vi "glueing_recovery.vi"() -> ()   [LabVIEW 2011]
panel:
  in  "OK Button 2":bool
  in  "Y to be glued (mm)":dbl
  in  "X to be glued (mm)":dbl
  in  "OK Button":bool
  in  "Motor":u16(ring) items=["X", "Y", "Z", "Gluer", "Spint"]
  in  "mm":dbl
  in  "KILL":bool
  in  "PAUSE":bool
  in  "RESUME":bool
  in  "QUIT":bool
  in  "zero Spint":bool
  out "output":string
  out "command":string
  in  "zero Gluer":bool
  in  "zero x":bool
  in  "zero y":bool
  # "Posiziono in zero"
  # "Movimentazione Motori"
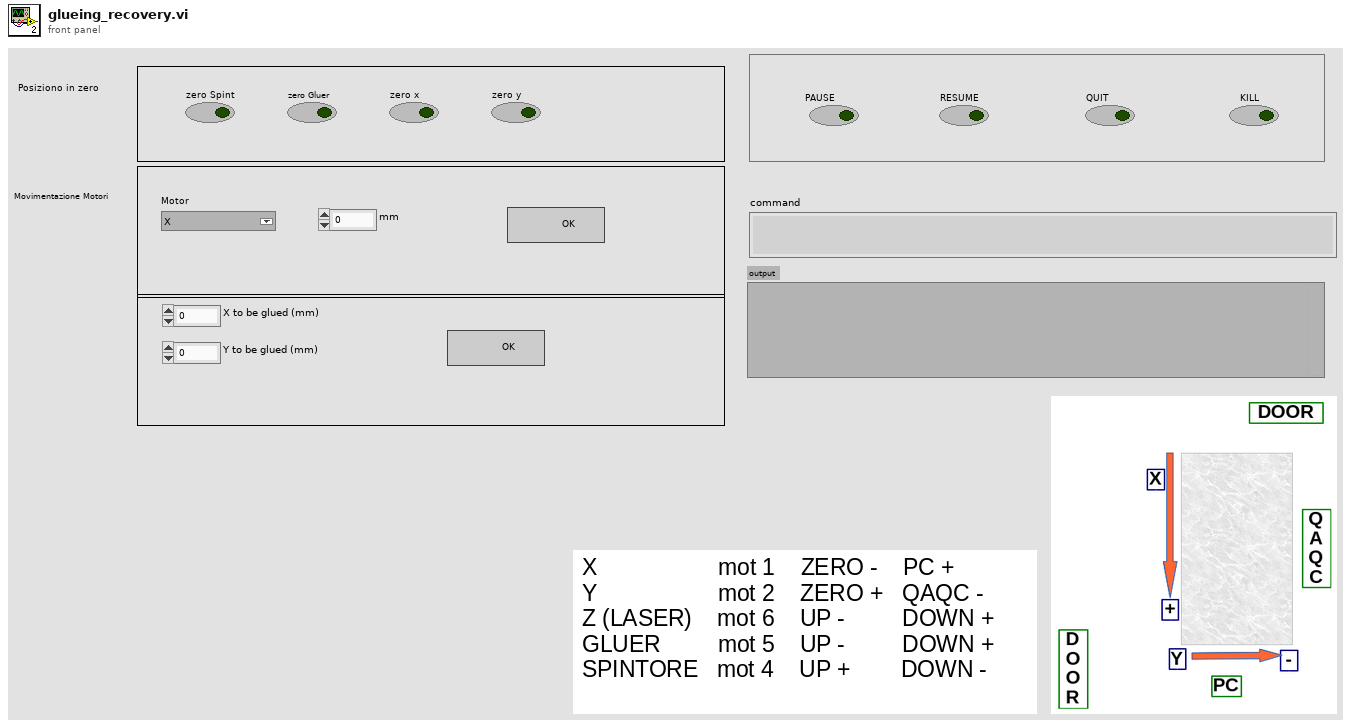
[diagram p1: front panel]
types:
  T1 = enum16{"open", "replace", "create", "open or create", "replace or create", "replace or create with confirmation"}
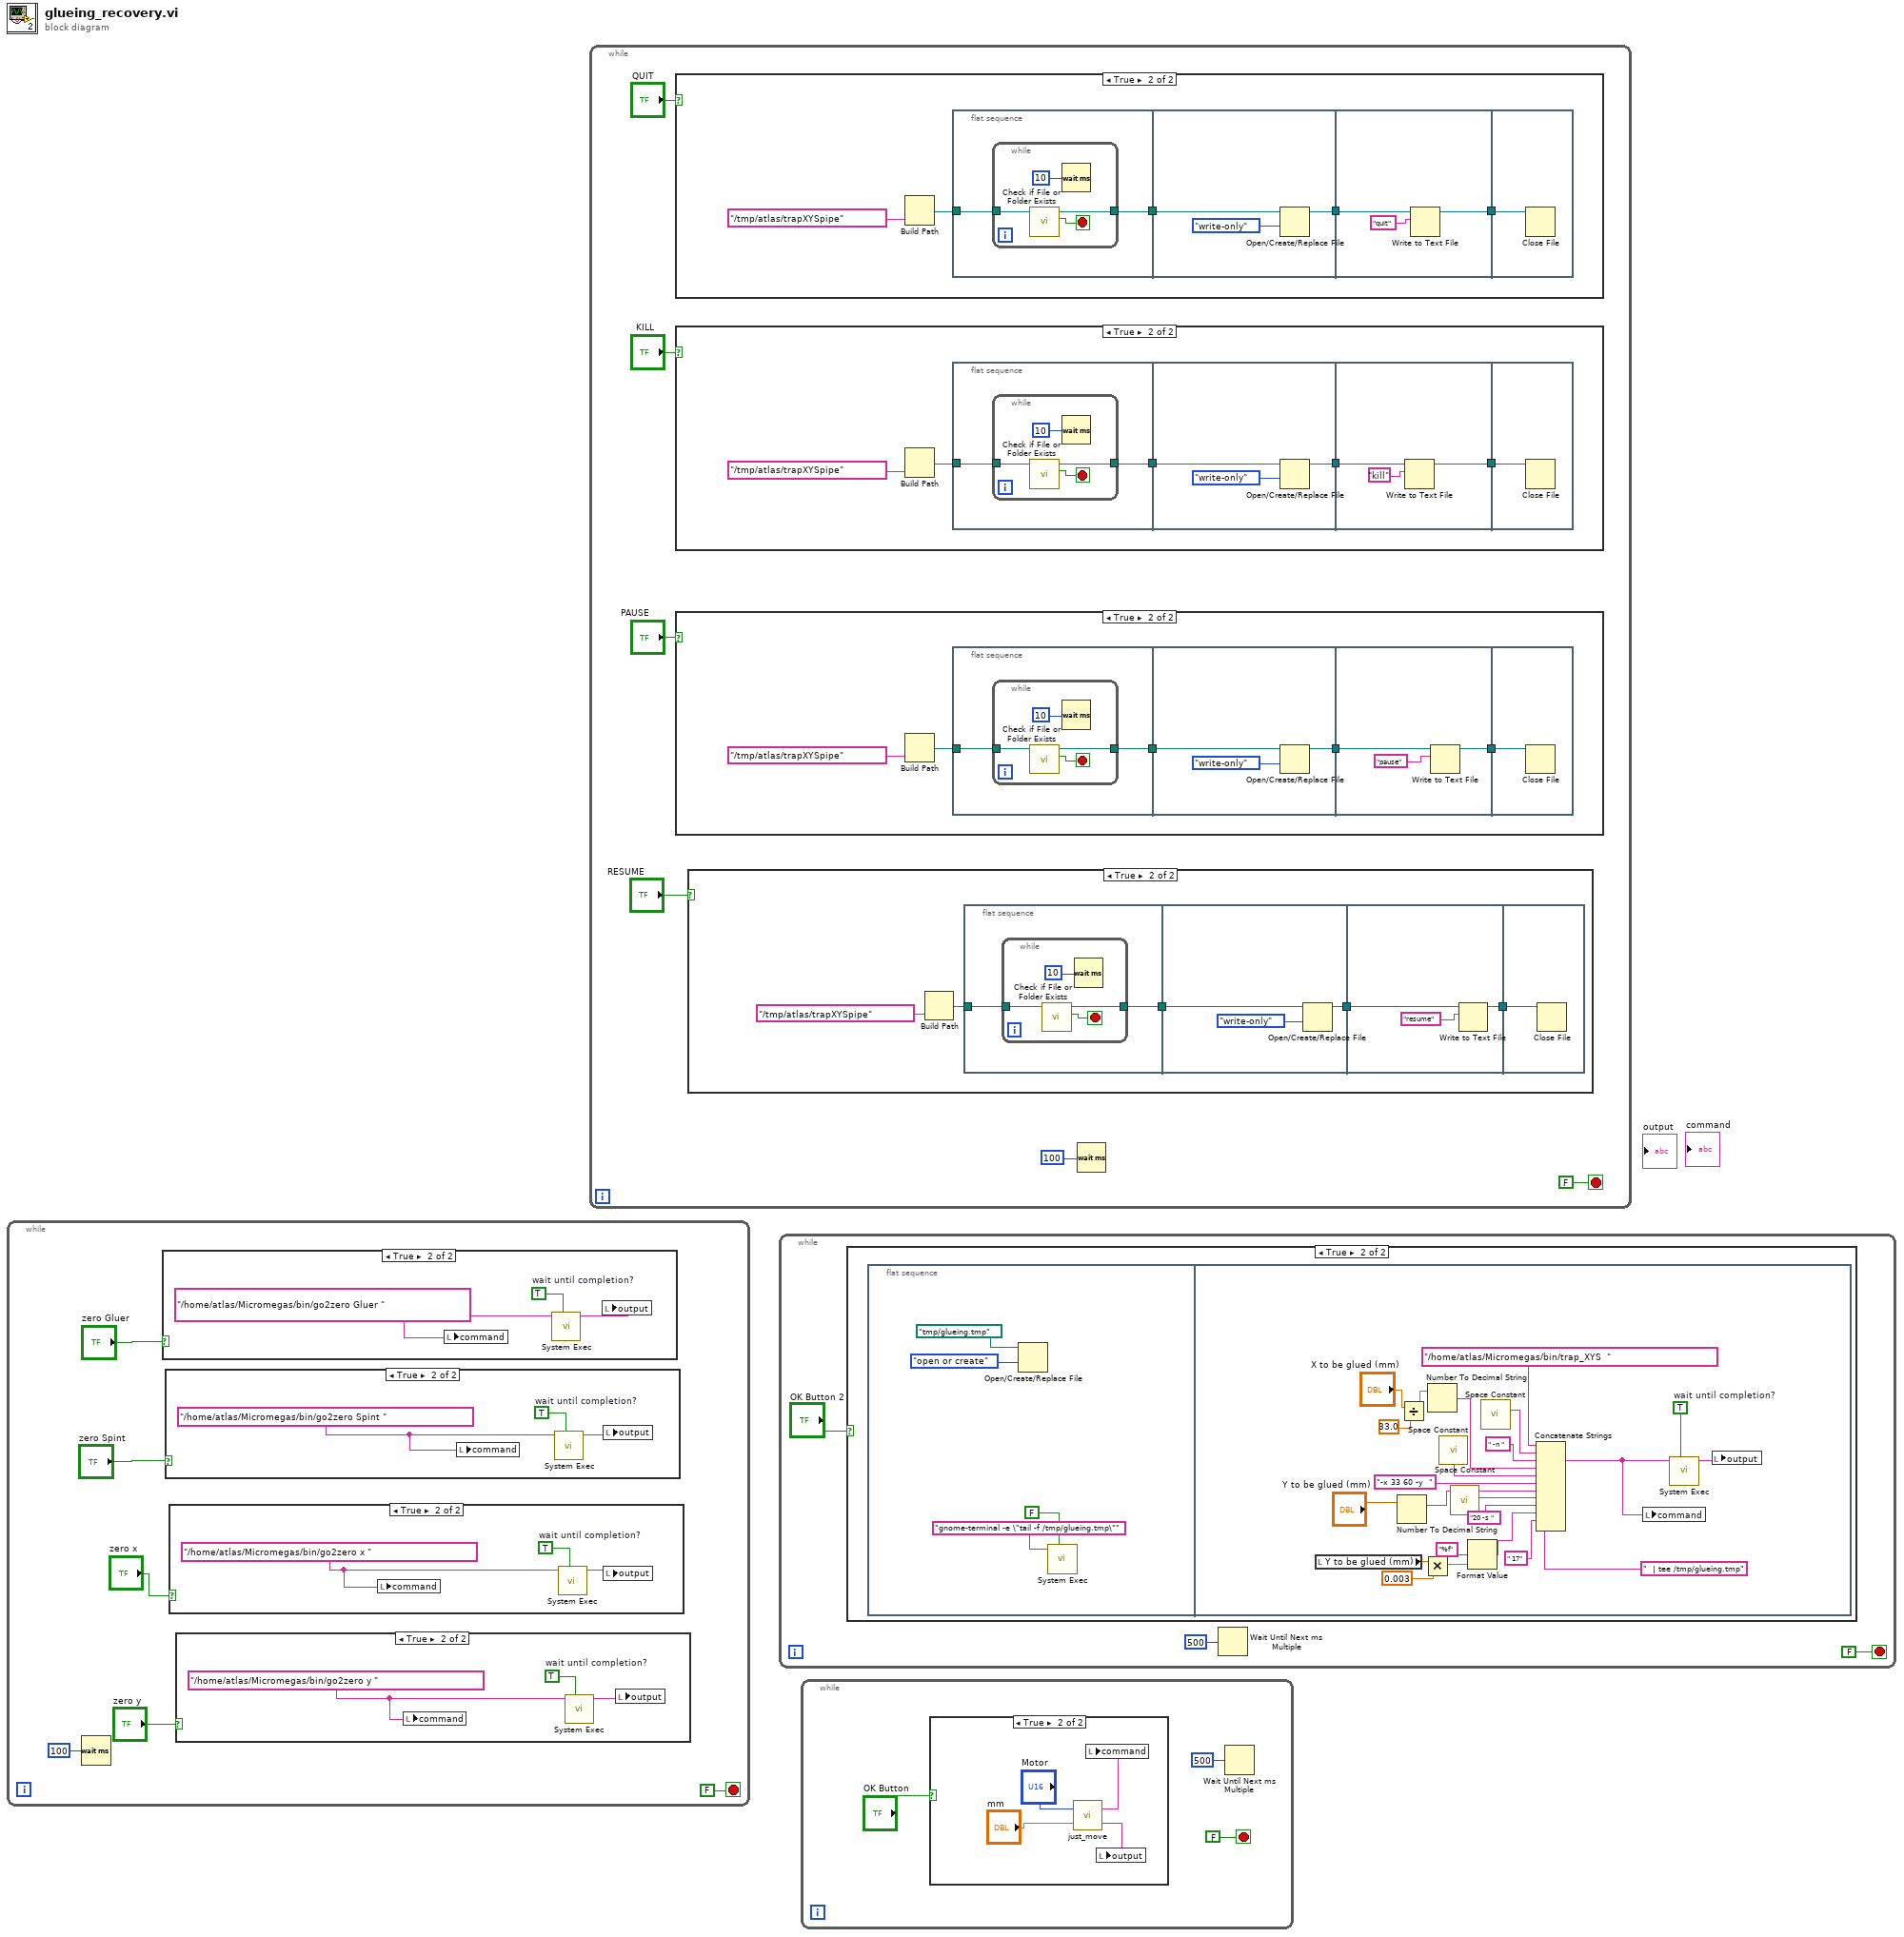
[diagram p0: block diagram]
diagram:
  n1 = while {
    stop <- FALSE stop-if-true
    n2 = Wait (ms)(milliseconds to wait=u32 100) -> ()  [unwired: 1 out]
    n3 = case shown="True" "zero Gluer" {
      frame False {
      }
      frame True {
        w17 = "/home/atlas/Micromegas/bin/go2zero Gluer " ("string")
        w18 = TRUE  # wait until completion?
        n4 = local write "command"(w17) -> ()
        n5 = call <vilib>:"System Exec.vi"("wait until completion? (T)"=w18, "command line"=w17) -> ("standard output"=w16:string)  [unwired: 6 in, 3 out]
        n6 = local write "output"(w16) -> ()
      }
    }
    n7 = case shown="True" "zero Spint" {
      frame False {
      }
      frame True {
        w7 = "/home/atlas/Micromegas/bin/go2zero Spint " ("string")
        w9 = TRUE  # wait until completion?
        n8 = local write "command"(w7) -> ()
        n9 = call <vilib>:"System Exec.vi"("wait until completion? (T)"=w9, "command line"=w7) -> ("standard output"=w8:string)  [unwired: 6 in, 3 out]
        n10 = local write "output"(w8) -> ()
      }
    }
    n11 = case shown="True" "zero x" {
      frame False {
      }
      frame True {
        w14 = "/home/atlas/Micromegas/bin/go2zero x " ("string")
        w15 = TRUE  # wait until completion?
        n12 = local write "command"(w14) -> ()
        n13 = call <vilib>:"System Exec.vi"("wait until completion? (T)"=w15, "command line"=w14) -> ("standard output"=w13:string)  [unwired: 6 in, 3 out]
        n14 = local write "output"(w13) -> ()
      }
    }
    n15 = case shown="True" "zero y" {
      frame False {
      }
      frame True {
        w11 = "/home/atlas/Micromegas/bin/go2zero y " ("string")
        w12 = TRUE  # wait until completion?
        n16 = local write "command"(w11) -> ()
        n17 = call <vilib>:"System Exec.vi"("wait until completion? (T)"=w12, "command line"=w11) -> ("standard output"=w10:string)  [unwired: 6 in, 3 out]
        n18 = local write "output"(w10) -> ()
      }
    }
  }
  n19 = while {
    stop <- FALSE stop-if-true
    n20 = case shown="True" "QUIT" {
      frame False {
      }
      frame True {
        n21 = Build Path(name or relative path="/tmp/atlas/trapXYSpipe" ("string")) -> (appended path=w79:path)  [unwired: 1 in]
        n22 = flat-sequence {
          tunnel: [w85] -> w83
          tunnel: w79 -> [w84]
          tunnel: w83 -> [w92]
          tunnel: [w90] -> w82
          tunnel: w82 -> [w95]
          tunnel: [w94] -> w81
          tunnel: w81 -> [w96]
          frame #0 {
            n23 = while {
              tunnel: [w87] -> w85
              tunnel: w84 -> [w86]
              stop <- w88 stop-if-true
              n24 = call <vilib>:"Check if File or Folder Exists.vi"("path"=w86) -> ("file or folder exists?"=w88:bool, "dup path"=w87:path)  [unwired: 8 in, 1 out]
              n25 = Wait (ms)(milliseconds to wait=u32 10) -> ()  [unwired: 1 out]
            }
          }
          frame #1 {
            n26 = Open/Create/Replace File(file path (use dialog)=w92, access (0:read/write)=enum16{"read/write", "read-only", "write-only"}."write-only") -> (refnum out=w90:refnum<file>)  [unwired: 4 in, 2 out]
          }
          frame #2 {
            n27 = Write to Text File(file (use dialog)=w95, text="quit") -> (refnum out=w94:refnum<file>)  [unwired: 2 in, 2 out]
          }
          frame #3 {
            n28 = Close File(refnum=w96) -> ()  [unwired: 1 in, 2 out]
          }
        }
      }
    }
    n29 = case shown="True" "KILL" {
      frame False {
      }
      frame True {
        n30 = Build Path(name or relative path="/tmp/atlas/trapXYSpipe" ("string")) -> (appended path=w43:path)  [unwired: 1 in]
        n31 = flat-sequence {
          tunnel: [w49] -> w47
          tunnel: w43 -> [w48]
          tunnel: w47 -> [w56]
          tunnel: [w54] -> w46
          tunnel: w46 -> [w59]
          tunnel: [w58] -> w45
          tunnel: w45 -> [w60]
          frame #0 {
            n32 = while {
              tunnel: [w51] -> w49
              tunnel: w48 -> [w50]
              stop <- w52 stop-if-true
              n33 = call <vilib>:"Check if File or Folder Exists.vi"("path"=w50) -> ("file or folder exists?"=w52:bool, "dup path"=w51:path)  [unwired: 8 in, 1 out]
              n34 = Wait (ms)(milliseconds to wait=u32 10) -> ()  [unwired: 1 out]
            }
          }
          frame #1 {
            n35 = Open/Create/Replace File(file path (use dialog)=w56, access (0:read/write)=enum16{"read/write", "read-only", "write-only"}."write-only") -> (refnum out=w54:refnum<file>)  [unwired: 4 in, 2 out]
          }
          frame #2 {
            n36 = Write to Text File(file (use dialog)=w59, text="kill") -> (refnum out=w58:refnum<file>)  [unwired: 2 in, 2 out]
          }
          frame #3 {
            n37 = Close File(refnum=w60) -> ()  [unwired: 1 in, 2 out]
          }
        }
      }
    }
    n38 = case shown="True" "PAUSE" {
      frame False {
      }
      frame True {
        n39 = Build Path(name or relative path="/tmp/atlas/trapXYSpipe" ("string")) -> (appended path=w25:path)  [unwired: 1 in]
        n40 = flat-sequence {
          tunnel: [w31] -> w29
          tunnel: w25 -> [w30]
          tunnel: w29 -> [w38]
          tunnel: [w36] -> w28
          tunnel: w28 -> [w41]
          tunnel: [w40] -> w27
          tunnel: w27 -> [w42]
          frame #0 {
            n41 = while {
              tunnel: [w33] -> w31
              tunnel: w30 -> [w32]
              stop <- w34 stop-if-true
              n42 = call <vilib>:"Check if File or Folder Exists.vi"("path"=w32) -> ("file or folder exists?"=w34:bool, "dup path"=w33:path)  [unwired: 8 in, 1 out]
              n43 = Wait (ms)(milliseconds to wait=u32 10) -> ()  [unwired: 1 out]
            }
          }
          frame #1 {
            n44 = Open/Create/Replace File(file path (use dialog)=w38, access (0:read/write)=enum16{"read/write", "read-only", "write-only"}."write-only") -> (refnum out=w36:refnum<file>)  [unwired: 4 in, 2 out]
          }
          frame #2 {
            n45 = Write to Text File(file (use dialog)=w41, text="pause") -> (refnum out=w40:refnum<file>)  [unwired: 2 in, 2 out]
          }
          frame #3 {
            n46 = Close File(refnum=w42) -> ()  [unwired: 1 in, 2 out]
          }
        }
      }
    }
    n47 = case shown="True" "RESUME" {
      frame False {
      }
      frame True {
        n48 = Build Path(name or relative path="/tmp/atlas/trapXYSpipe" ("string")) -> (appended path=w61:path)  [unwired: 1 in]
        n49 = flat-sequence {
          tunnel: [w67] -> w65
          tunnel: w61 -> [w66]
          tunnel: w65 -> [w74]
          tunnel: [w72] -> w64
          tunnel: w64 -> [w77]
          tunnel: [w76] -> w63
          tunnel: w63 -> [w78]
          frame #0 {
            n50 = while {
              tunnel: [w69] -> w67
              tunnel: w66 -> [w68]
              stop <- w70 stop-if-true
              n51 = call <vilib>:"Check if File or Folder Exists.vi"("path"=w68) -> ("file or folder exists?"=w70:bool, "dup path"=w69:path)  [unwired: 8 in, 1 out]
              n52 = Wait (ms)(milliseconds to wait=u32 10) -> ()  [unwired: 1 out]
            }
          }
          frame #1 {
            n53 = Open/Create/Replace File(file path (use dialog)=w74, access (0:read/write)=enum16{"read/write", "read-only", "write-only"}."write-only") -> (refnum out=w72:refnum<file>)  [unwired: 4 in, 2 out]
          }
          frame #2 {
            n54 = Write to Text File(file (use dialog)=w77, text="resume") -> (refnum out=w76:refnum<file>)  [unwired: 2 in, 2 out]
          }
          frame #3 {
            n55 = Close File(refnum=w78) -> ()  [unwired: 1 in, 2 out]
          }
        }
      }
    }
    n56 = Wait (ms)(milliseconds to wait=100) -> ()  [unwired: 1 out]
  }
  n57 = while {
    stop <- FALSE stop-if-true
    n58 = case shown="True" "OK Button 2" {
      frame False {
      }
      frame True {
        n59 = flat-sequence {
          frame #0 {
            n60 = Open/Create/Replace File(file path (use dialog)=path "/tmp/glueing.tmp", operation (0:open)=T1."open or create") -> ()  [unwired: 4 in, 3 out]
            n61 = call <vilib>:"System Exec.vi"("wait until completion? (T)"=FALSE, "command line"="gnome-terminal -e \"tail -f /tmp/glueing.tmp\"" ("logwindow")) -> ()  [unwired: 6 in, 4 out]
          }
          frame #1 {
            w126 = TRUE  # wait until completion?
            n62 = local read "Y to be glued (mm)"() -> (w112:dbl)
            n63 = Number To Decimal String(number="Y to be glued (mm)") -> (decimal integer string=w108:string)  [unwired: 1 in]
            n64 = Divide(x="X to be glued (mm)", y=33.0) -> (x/y=w106:dbl)
            n65 = Multiply(x=w112, y=0.003) -> (x*y=w109:dbl)
            n66 = Number To Decimal String(number=w106) -> (decimal integer string=w105:string)  [unwired: 1 in]
            n67 = call <vilib>:"Space Constant.vi"() -> ("String"=w115:string)
            n68 = call <vilib>:"Space Constant.vi"() -> ("String"=w114:string)
            n69 = Format Value(format string="%f", value (0)=w109) -> (output string=w110:string)  [unwired: 1 in]
            n70 = call <vilib>:"Space Constant.vi"() -> ("String"=w120:string)
            n71 = Concatenate Strings("/home/atlas/Micromegas/bin/trap_XYS  " ("string"), w120, " -n " ("string"), w105, w115, "-x 33 60 -y  " ("string"), w108, w114, "20 -s " ("string"), w110, " 17" ("string"), "  | tee /tmp/glueing.tmp" ("string")) -> (w104:string)
            n72 = local write "command"(w104) -> ()
            n73 = call <vilib>:"System Exec.vi"("wait until completion? (T)"=w126, "command line"=w104) -> ("standard output"=w123:string)  [unwired: 6 in, 3 out]
            n74 = local write "output"(w123) -> ()
          }
        }
      }
    }
    n75 = Wait Until Next ms Multiple(millisecond multiple=u32 500) -> ()  [unwired: 1 out]
  }
  n76 = while {
    stop <- FALSE stop-if-true
    n77 = case shown="True" "OK Button" {
      frame False {
      }
      frame True {
        n78 = call "just_move.vi"("mm"="mm", "Motor"="Motor") -> ("output"=w133:string, "command"=w132:string)
        n79 = local write "command"(w132) -> ()
        n80 = local write "output"(w133) -> ()
      }
    }
    n81 = Wait Until Next ms Multiple(millisecond multiple=u32 500) -> ()  [unwired: 1 out]
  }
